vi "linear interpolation - bb - complex.vi"(0 "Array":cdb[](array[numeric]), 11 "center":i32=-1) -> (2 "bb":dbl, 3 "directed sigma":dbl, 4 "left":cdb, 6 "center":cdb, 8 "right":cdb, 10 "mean":cdb, 12 "intercept":cdb, 14 "slope":cdb, 15 "interpolated average":cdb)   [LabVIEW 2015]
panel:
  out "sum z_n":cdb
  out "sum n z_n":cdb
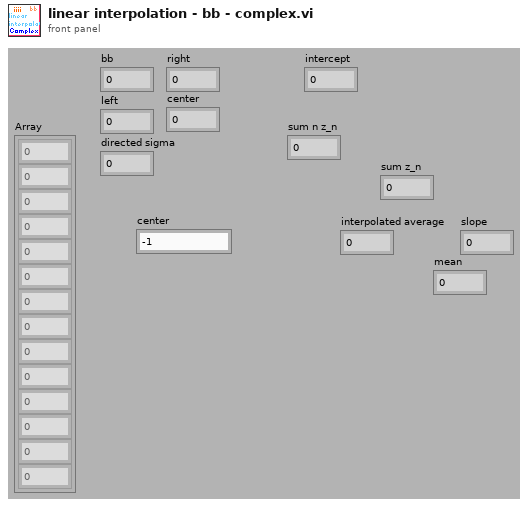
[diagram p1: front panel]
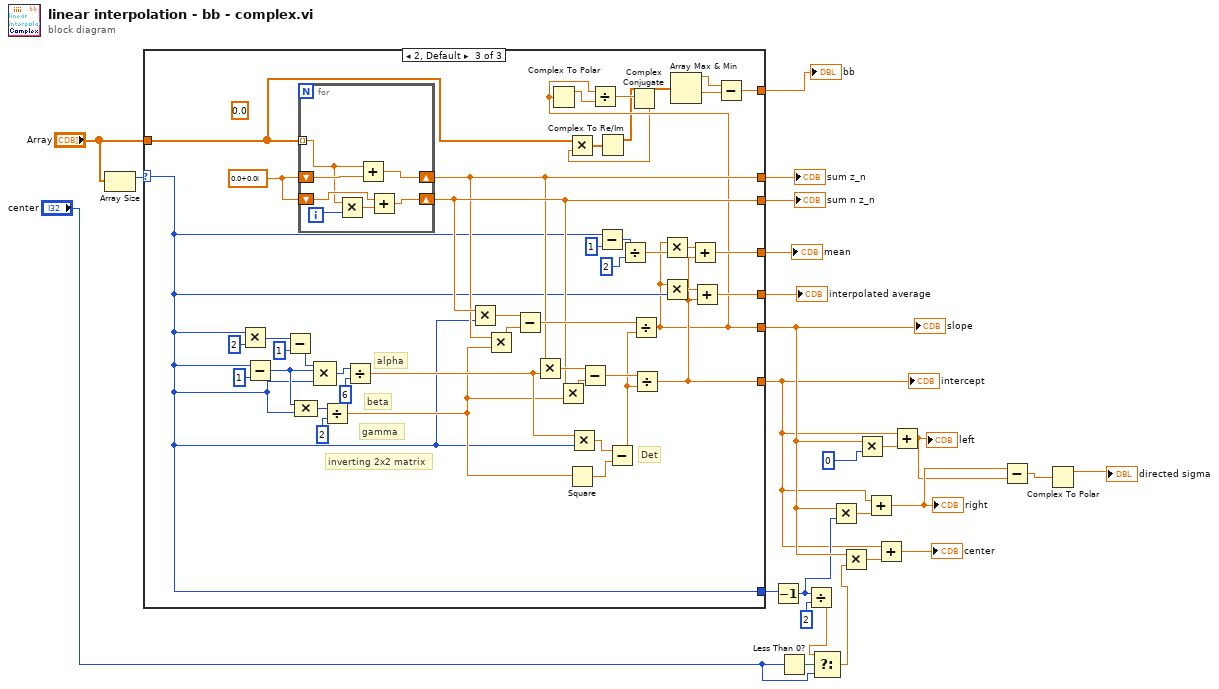
[diagram p0: block diagram]
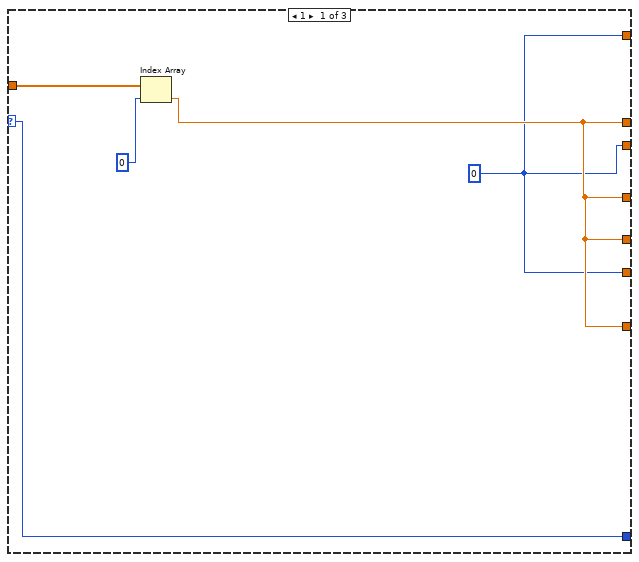
[diagram p2: hidden frame]
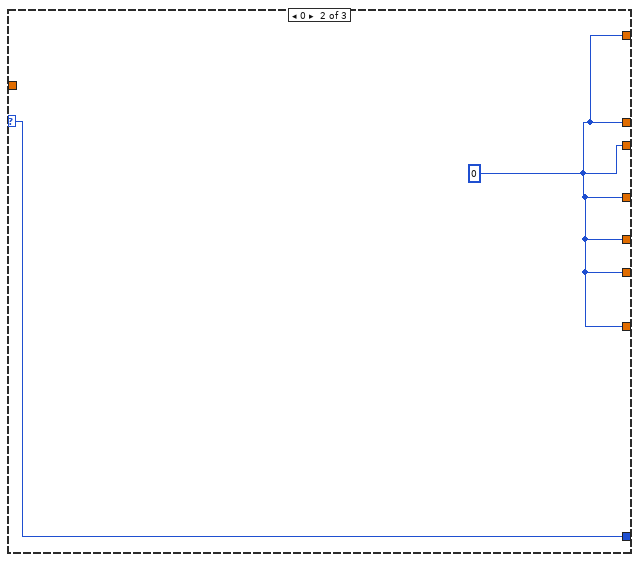
[diagram p3: hidden frame]
diagram:
  n1 = Array Size(array="Array") -> (size(s)=w20:i32)
  n2 = case shown="2, Default" w20 {
    selector: w20 -> [w27 w32 w43]
    tunnel: [w28 w31 w49] -> w10
    tunnel: [w26 w31 w41] -> w13
    tunnel: [w28 w31 w48] -> w25
    tunnel: [w28 w31 w47] -> w24
    tunnel: [w28 w31 w44] -> w23
    tunnel: [w26 w31 w46] -> w22
    tunnel: "Array" -> [w30 _ w39]
    tunnel: [w27 w32 w43] -> w14
    tunnel: [w26 w31 w33] -> w1
    frame 1 {
      w26 = 0 ("index")
      n3 = Index Array(array=w30, index=0) -> (element=w28:cdb)
    }
    frame 0 {
      w31 = 0 ("index")
    }
    frame 2, Default {
      (unwired) 0.0
      w45 = cdb 0.0+0.0i
      # "inverting 2x2 matrix"
      # "Det"
      # "beta"
      # "gamma"
      # "alpha"
      n4 = Multiply(x=w43, y=2 ("n")) -> (x*y=w73:i32)
      n5 = Subtract(x=w43, y=1 ("n")) -> (x-y=w69:i32)
      n6 = Subtract(x=w73, y=1 ("n")) -> (x-y=w72:i32)
      n7 = Compound Arithmetic op=MULTIPLY(w69, w43) -> (w67:i32)
      n8 = for {
        tunnel: w39 -> [w77] mode=indexing
        shift-right: [w83] -> w44
        shift-left: w45 -> [w82]
        shift-right: [w80] -> w46
        shift-left: w45 -> [w78]
        i -> [w79]
        n9 = Multiply(x=w77, y=w79) -> (x*y=w81:cdb)
        n10 = Add(x=w77, y=w82) -> (x+y=w83:cdb)
        n11 = Add(x=w78, y=w81) -> (x+y=w80:cdb)
      }
      n12 = Compound Arithmetic op=MULTIPLY(w72, w69, w43) -> (w71:i32)
      n13 = Divide(x=w67, y=2 ("n")) -> (x/y=w58:dbl)
      n14 = Divide(x=w71, y=6 ("n")) -> (x/y=w59:dbl)
      n15 = Multiply(x=w46, y=w43) -> (x*y=w63:cdb)
      n16 = Multiply(x=w44, y=w58) -> (x*y=w64:cdb)
      n17 = Subtract(x=w63, y=w64) -> (x-y=w62:cdb)
      n18 = Multiply(x=w44, y=w59) -> (x*y=w60:cdb)
      n19 = Multiply(x=w46, y=w58) -> (x*y=w61:cdb)
      n20 = Square(x=w58) -> (x^2=w65:dbl)
      n21 = Multiply(x=w59, y=w43) -> (x*y=w66:dbl)
      n22 = Subtract(x=w60, y=w61) -> (x-y=w57:cdb)
      n23 = Subtract(x=w43, y=1 ("n")) -> (x-y=w54:i32)
      n24 = Subtract(x=w66, y=w65) -> (x-y=w56:dbl)
      n25 = Divide(x=w54, y=2 ("n")) -> (x/y=w52:dbl)
      n26 = Divide(x=w62, y=w56) -> (x/y=w41:cdb)
      n27 = Complex To Polar(r * e^(i*theta)=w41) -> (r=w42:dbl)  [unwired: 1 out]
      n28 = Divide(x=w41, y=w42) -> (x/y=w40:cdb)
      n29 = Complex Conjugate(1:w40) -> (0:w38:cdb)
      n30 = Multiply(x=w39, y=w38) -> (x*y=w37:cdb[])
      n31 = Complex To Re/Im(x + iy=w37) -> (x=w36:dbl[])  [unwired: 1 out]
      n32 = Divide(x=w57, y=w56) -> (x/y=w49:cdb)
      n33 = Multiply(x=w41, y=w52) -> (x*y=w51:cdb)
      n34 = Multiply(x=w41, y=w43) -> (x*y=w50:cdb)
      n35 = Array Max & Min(array=w36) -> (max value=w35:dbl, min value=w34:dbl)  [unwired: 2 out]
      n36 = Add(x=w51, y=w49) -> (x+y=w47:cdb)
      n37 = Add(x=w50, y=w49) -> (x+y=w48:cdb)
      n38 = Subtract(x=w35, y=w34) -> (x-y=w33:dbl)
    }
  }
  "interpolated average" <- w25
  "slope" <- w13
  "mean" <- w24
  "intercept" <- w10
  "sum n z_n" <- w22
  "sum z_n" <- w23
  "bb" <- w1
  n39 = Decrement(x=w14) -> (x-1=w12:i32)
  n40 = Less Than 0?(x="center") -> (x < 0?=w9:bool)
  n41 = Divide(x=w12, y=2 ("n")) -> (x/y=w8:dbl)
  n42 = Select(t=w8, s=w9, f="center") -> (s? t:f=w6:dbl)
  n43 = Multiply(x=w13, y=w12) -> (x*y=w17:cdb)
  n44 = Multiply(x=w13, y=w6) -> (x*y=w16:cdb)
  n45 = Multiply(x=w13, y=0 ("n")) -> (x*y=w18:cdb)
  n46 = Add(x=w10, y=w17) -> (x+y=w5:cdb)
  "right" <- w5
  n47 = Add(x=w10, y=w16) -> (x+y=→"center":cdb)
  n48 = Add(x=w10, y=w18) -> (x+y=w4:cdb)
  "left" <- w4
  n49 = Subtract(x=w5, y=w4) -> (x-y=w3:cdb)
  n50 = Complex To Polar(r * e^(i*theta)=w3) -> (r=→"directed sigma":dbl)  [unwired: 1 out]
